vi "CTRE_PigeonIMU_GetBiasedMagnetometer.vi"(8 "error in (no error)":errorcluster, 11 "PigeonIMUDevRef":T1={"DeviceStatus"={"status"=FALSE, "code"=0, "source"=""}, "Device Number"=0, "Type"=352321536, "Device ID"=0, "Handle"=0, "UsageFrame"=0, "Library Path"=path ""} {"Type" items=["CAN"=352321536, "TalonSRX"=33554432]}) -> (0 "error out":errorcluster, 2 "Biased Magnetometer":cluster{"X":i16, "Y":i16, "Z":i16}, 3 "PigeonIMUDevRef":T1={"DeviceStatus"={"status"=FALSE, "code"=0, "source"=""}, "Device Number"=0, "Type"=352321536, "Device ID"=0, "Handle"=0, "UsageFrame"=0, "Library Path"=path ""} {"Type" items=["CAN"=352321536, "TalonSRX"=33554432]})   [LabVIEW 2016]
uses:
  <vilib>/Rock Robotics/WPI/ThirdParty/Sensors/Pigeon IMU/CTRE_PigeonIMU_DeviceRef.ctl
  <vilib>/Rock Robotics/WPI/ThirdParty/Sensors/Pigeon IMU/CTRE_PigeonIMU_ConnectionType.ctl
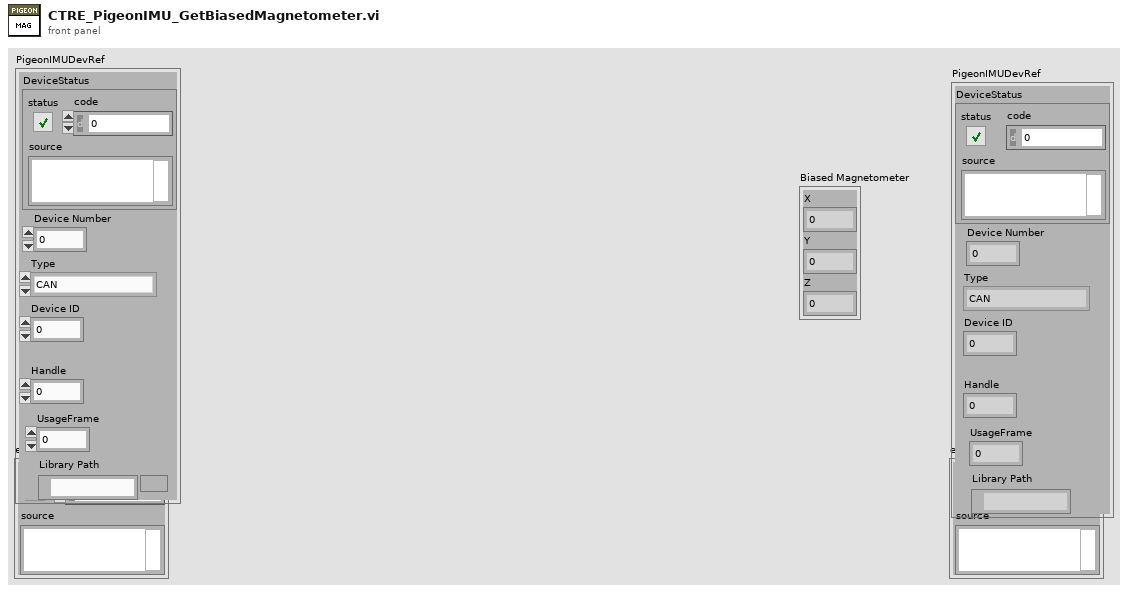
[diagram p1: front panel]
types:
  T1 = typedef "CTRE_PigeonIMU_DeviceRef.ctl" = cluster{"DeviceStatus":errorcluster, "Device Number":u8, "Type":T2, "Device ID":u32, "Handle":u64, "UsageFrame":u32, "Library Path":path}
  T2 = typedef "CTRE_PigeonIMU_ConnectionType.ctl" = u32
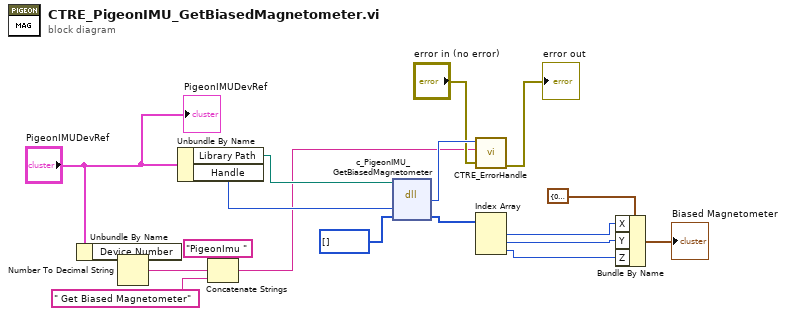
[diagram p0: block diagram]
diagram:
  n1 = Unbundle By Name("PigeonIMUDevRef") -> ("Device Number"=w6:u8)
  n2 = Number To Decimal String(number=w6) -> (decimal integer string=w5:string)  [unwired: 1 in]
  n3 = Unbundle By Name("PigeonIMUDevRef") -> ("Library Path"=w18:path, "Handle"=w17:u64)
  n4 = Concatenate Strings("PigeonImu " ("string"), w5, " Get Biased Magnetometer" ("string")) -> (w1:string)
  n5 = dll-call lib="?" fn="c_PigeonIMU_GetBiasedMagnetometer"(path in=w18, "handle"=w17, "bm_xyz"=i16[] [] ("ba_xyz")) -> ("return type"=w9:i32, "bm_xyz"=w16:i16[])  [unwired: 3 in, 2 out]
  n6 = call <vilib>:"CTRE_ErrorHandle.vi"("error in"="error in (no error)", "origin"=w1, "code"=w9) -> ("error out"=→"error out":errorcluster)  [unwired: 8 in]
  n7 = Index Array(array=w16) -> (element #1=w15:i16, element #2=w14:i16, element #3=w13:i16)  [unwired: 3 in]
  n8 = Bundle By Name(cluster=cluster{"X":i16, "Y":i16, "Z":i16} {"X"=0, "Y"=0, "Z"=0} ("Biased"), "X"=w15, "Y"=w14, "Z"=w13) -> (→"Biased Magnetometer":cluster{"X":i16, "Y":i16, "Z":i16})
  "PigeonIMUDevRef" <- "PigeonIMUDevRef"
